vi "Send Command.vi"(7 "Timeout (100 ms)":i32=100, 8 "Error In":errorcluster, 9 "ARGS":u8[](array[numeric]), 10 "CMD":u16, 11 "LINX Device Config":T1) -> (0 "Error Out":errorcluster, 1 "Status":u8, 2 "Response":u8[](array[numeric]), 3 "LINX Device Config":T1)   [LabVIEW 2018, in "LVH-LINX.lvlib" / "Device.lvlib"]
doc: "Send a packet to the LINX device and return the LINX device response packet."
uses:
  Device.lvlib
  Type Defs/LINX Device Config.ctl
  Type Defs/Interface.ctl
  Type Defs/TCP Config.ctl
  Type Defs/Device Family.ctl
  Type Defs/Error Type.ctl
  LVH-LINX.lvlib
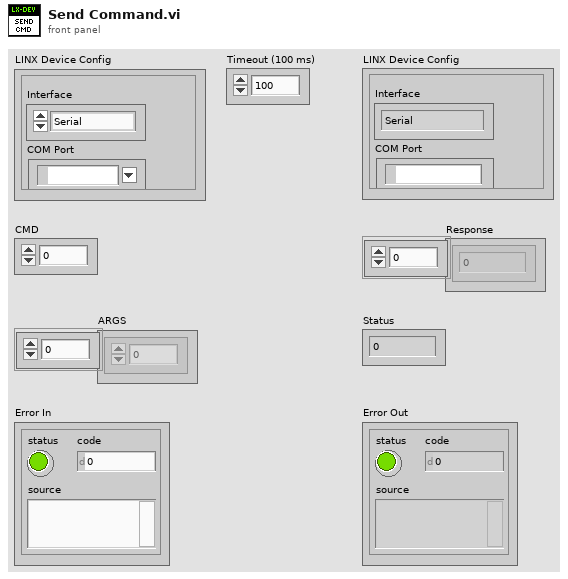
[diagram p1: front panel]
types:
  T1 = typedef "LVH-LINX.lvlib/Device.lvlib/LINX Device Config.ctl" = cluster{"Interface":T2, "COM Port":refnum<visa-resource-name>, "TCP Configuration":T3, "Device Family":T4, "Device ID":u8, "Device Name":string, "TCP Ref":refnum<k5>}
  T2 = typedef "LVH-LINX.lvlib/Interface.ctl" = enum16{"Serial", "TCP"}
  T3 = typedef "LVH-LINX.lvlib/Device.lvlib/TCP Config.ctl" = cluster{"IP Address":string, "Port":u16}
  T4 = typedef "LVH-LINX.lvlib/Device Family.ctl" = enum8{"National Instruments", "Digilent", "Arduino"}
  T5 = typedef "LVH-LINX.lvlib/Error Type.ctl" = enum16{"Unknown", "Timeout", "Corrupt Return Packet", "Unable To Connect", "Command Not Supported", "Channel DNE", "Invalid COM Config"}
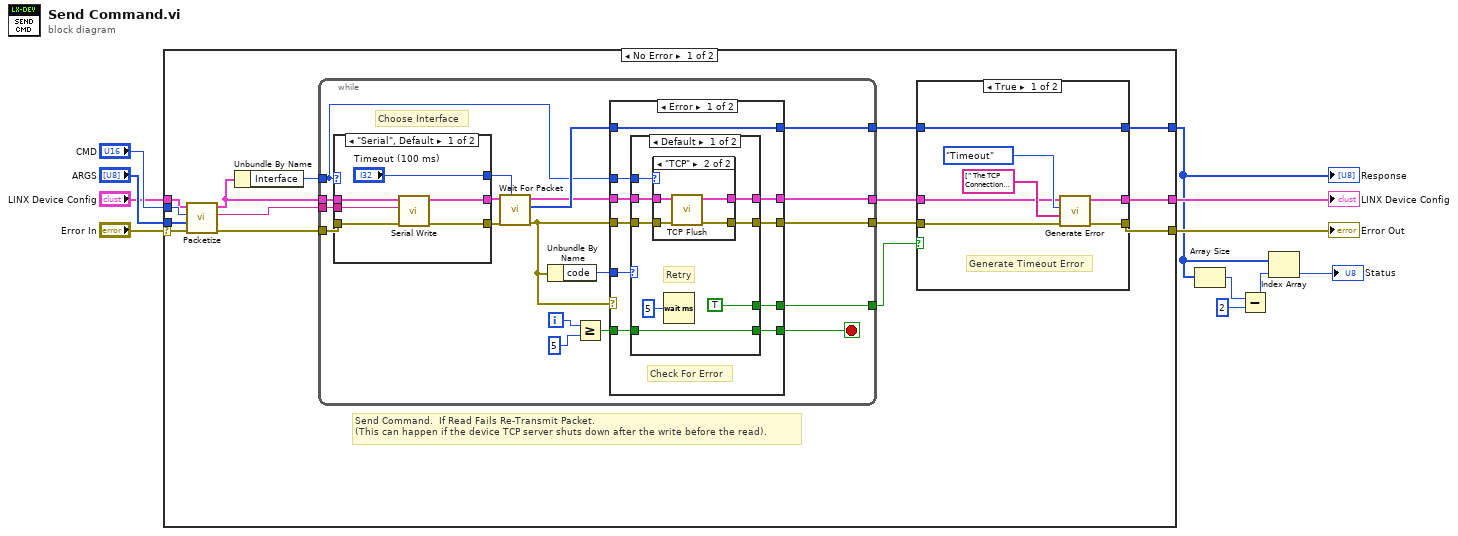
[diagram p0: block diagram]
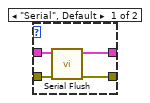
[diagram p3: hidden frame]
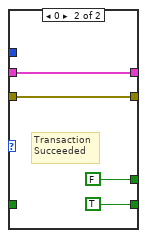
[diagram p4: hidden frame]
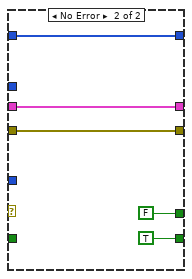
[diagram p5: hidden frame]
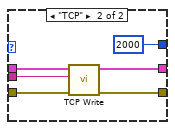
[diagram p6: hidden frame]
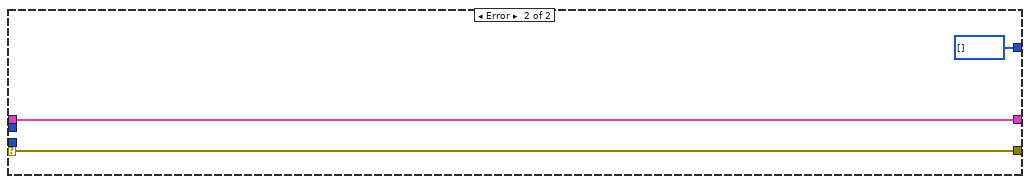
[diagram p7: hidden frame]
diagram:
  n1 = case shown="No Error" "Error In" {
    selector: "Error In" -> [w13 w103]
    tunnel: "ARGS" -> [w24 _]
    tunnel: "CMD" -> [w23 _]
    tunnel: "LINX Device Config" -> [w20 w105]
    tunnel: [w19 w105] -> w8
    tunnel: [w18 w103] -> w7
    tunnel: [w15 u8[] [] ("Packet")] -> w5
    frame No Error {
      # "Send Command.  If Read Fails Re-Transmit Packet.\n(This can happen if the device TCP server shuts down after the write before the read)."
      n2 = call "Packetize.vi"("Error In"=w13, "ARGS"=w24, "CMD"=w23, "LINX Device Config"=w20) -> ("Error Out"=w26:errorcluster, "Packet"=w25:string, "LINX Decice Config"=w22:T1)  [unwired: 5 in]
      n3 = Unbundle By Name(w22) -> ("Interface"=w21:T2)
      n4 = while {
        tunnel: w26 -> [w55]
        tunnel: w25 -> [w54]
        tunnel: w22 -> [w53]
        tunnel: w21 -> [w37]
        tunnel: [w42] -> w14
        tunnel: [w46] -> w17
        tunnel: [w39] -> w16
        tunnel: [w43] -> w12
        i -> [w50]
        stop <- w45 stop-if-true
        # "Choose Interface"
        n5 = case shown="\"Serial\", Default" w37 {
          tunnel: w53 -> [w95 w100]
          tunnel: w55 -> [w96 w101]
          tunnel: [w92 w98] -> w52
          tunnel: [w93 w99] -> w51
          tunnel: w54 -> [w94 w102]
          tunnel: ["Timeout (100 ms)" 2000 ("Timeout (100 ms)")] -> w48
          frame "Serial", Default {
            n6 = call "Serial Write.vi"("Error In"=w96, "Data"=w94, "LINX Device Config"=w95) -> ("Error Out"=w92:errorcluster, "LINX Device Config"=w93:T1)  [unwired: 7 in]
          }
          frame "TCP" {
            n7 = call "TCP Write.vi"("Error In"=w101, "Packet"=w102, "LINX Decice Config"=w100) -> ("Error Out"=w98:errorcluster, "LINX Decice Config"=w99:T1)  [unwired: 7 in]
          }
        }
        n8 = call "Wait For Packet.vi"("Timeout (100 ms)"=w48, "Error In"=w52, "LINX Device Config"=w51) -> ("Error Out"=w38:errorcluster, "Packet"=w41:u8[], "LINX Device Config"=w40:T1)  [unwired: 6 in]
        n9 = Unbundle By Name(w38) -> ("code"=w47:i32)
        n10 = Greater Or Equal?(x=w50, y=5) -> (x >= y?=w44:bool)
        n11 = case shown="Error" w38 {
          tunnel: w47 -> [w65 _]
          tunnel: [w64 w90] -> w46
          tunnel: [w63 TRUE] -> w45
          tunnel: w44 -> [w62 _]
          tunnel: [w61 FALSE] -> w43
          tunnel: [w60 w86] -> w42
          tunnel: w41 -> [w60 w86]
          tunnel: w40 -> [w59 w87]
          tunnel: [w58 w87] -> w39
          tunnel: w38 -> [w57 w90]
          tunnel: w37 -> [w56 _]
          frame Error {
            # "Check For Error"
            n12 = case shown="Default" w65 {
              tunnel: [w68 w85] -> w64
              tunnel: [w73 TRUE] -> w63
              tunnel: w62 -> [w73 _]
              tunnel: [TRUE FALSE] -> w61
              tunnel: w59 -> [w70 w82]
              tunnel: [w69 w82] -> w58
              tunnel: w57 -> [w67 w85]
              tunnel: w56 -> [w66 _]
              frame Default {
                # "Retry"
                n13 = case shown="\"TCP\"" w66 {
                  tunnel: w70 -> [w77 w81]
                  tunnel: [w76 w80] -> w69
                  tunnel: [w75 w79] -> w68
                  tunnel: w67 -> [w74 w78]
                  frame "Serial", Default {
                    n14 = call "Serial Flush.vi"("Error In"=w74, "LINX Device Config"=w77) -> ("Error Out"=w75:errorcluster, "LINX Device Config"=w76:T1)  [unwired: 8 in]
                  }
                  frame "TCP" {
                    n15 = call "TCP Flush.vi"("Error In"=w78, "LINX Device Config"=w81) -> ("Error Out"=w79:errorcluster, "LINX Device Config"=w80:T1)  [unwired: 7 in, 1 out]
                  }
                }
                n16 = Wait (ms)(milliseconds to wait=u32 5) -> ()  [unwired: 1 out]
              }
              frame 0 {
                # "Transaction \nSucceeded"
              }
            }
          }
          frame No Error {
          }
        }
      }
      n17 = case shown="True" w12 {
        tunnel: [w33 w34] -> w18
        tunnel: [w30 w35] -> w19
        tunnel: w17 -> [w29 w34]
        tunnel: w16 -> [w28 w35]
        tunnel: [w27 w36] -> w15
        tunnel: w14 -> [w27 w36]
        frame True {
          # "Generate Timeout Error"
          n18 = call "Generate Error.vi"("Error In"=w29, "Arguments"=string[] [" The TCP Connection Was Refused."], "Error Type"=Error_Type."Timeout", "LINX Device Config"=w28) -> ("Error Out"=w33:errorcluster, "LINX Device Config"=w30:T1)  [unwired: 6 in]
        }
        frame False {
          # "Send/Rec Successful\nNo Error"
        }
      }
    }
    frame Error {
    }
  }
  "Error Out" <- w7
  "Response" <- w5
  "LINX Device Config" <- w8
  n19 = Array Size(array=w5) -> (size(s)=w4:i32)
  n20 = Subtract(x=w4, y=2 ("x")) -> (x-y=w3:i32)
  n21 = Index Array(array=w5, index=w3) -> (element=→"Status":u8)
